vi "Aspect Ratio Ball.vi"(10 "Circularity":dbl, 11 "Compactness":dbl) -> (3 "Score":dbl)   [LabVIEW 2020]
doc: "This VI compares the calculated diameter and convex hull area to compare this shape to a half-hexagon."
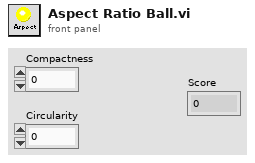
[diagram p1: front panel]
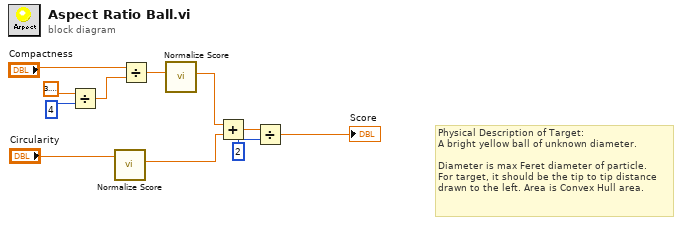
[diagram p0: block diagram]
diagram:
  # "Physical Description of Target:\nA bright yellow ball of unknown diameter.\n\nDiameter is max Feret diameter of particle.\nFor target, it should be the tip to tip distance\ndrawn to the left. Area is Convex Hull area."
  n1 = Divide(x=3.141592653589793, y=4) -> (x/y=w8:dbl)
  n2 = call "Normalize Score.vi"("Value"="Circularity") -> ("Score"=w3:dbl)  [unwired: 10 in]
  n3 = Divide(x="Compactness", y=w8) -> (x/y=w6:dbl)
  n4 = call "Normalize Score.vi"("Value"=w6) -> ("Score"=w2:dbl)  [unwired: 10 in]
  n5 = Add(x=w2, y=w3) -> (x+y=w4:dbl)
  n6 = Divide(x=w4, y=2) -> (x/y=→"Score":dbl)
